vi "Pointer.Read (1D DBL).vi"(8 "error in (no error)":errorcluster, 10 "count":i32, 11 "pointer in":u64) -> (0 "error out":errorcluster, 2 "values":dbl[](array[numeric]), 3 "pointer out":u64)   [LabVIEW 2016, in "VeriStand Data.lvlib"]
doc: "Reads a number of values, specified by <B>count</B>, from the provided <B>pointer</B>."
uses:
  VeriStand Data.lvlib
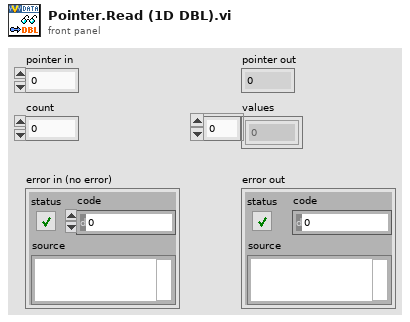
[diagram p1: front panel]
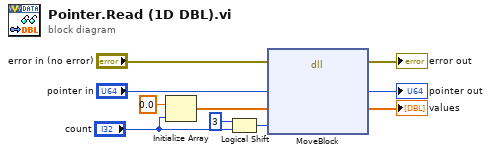
[diagram p0: block diagram]
diagram:
  n1 = Initialize Array(0.0 ("element"), "count") -> (w2:dbl[])
  n2 = Logical Shift(y=i16 3, x="count") -> (x << y=w4:i32)
  n3 = dll-call lib="LabVIEW" fn="MoveBlock"(error in="error in (no error)", "ps"="pointer in", "pd"=w2, "size"=w4) -> (error out=→"error out":errorcluster, "ps"=→"pointer out":u64, "pd"=→"values":dbl[])  [unwired: 4 in, 1 out]
